vi "solar_misc CPU Usage.vi"(8 "error in (no error)":errorcluster, 9 "Close Refnums? (F)":bool) -> (0 "error out":errorcluster, 2 "Processor CPU Usage (%)":dbl[](array[numeric]), 3 "Total CPU Usage (%)":dbl)   [LabVIEW 2018]
doc: "This returns the CPU utilization in percent for each processor using the .NET System.Diagnostics.PerformanceCounter API."
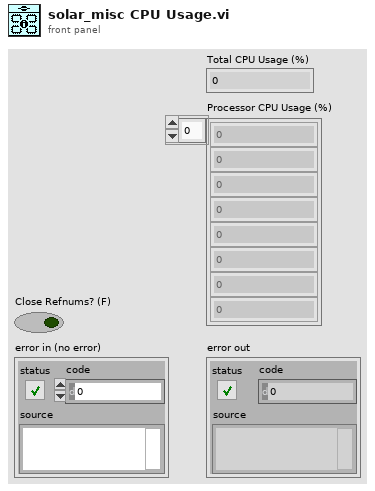
[diagram p1: front panel]
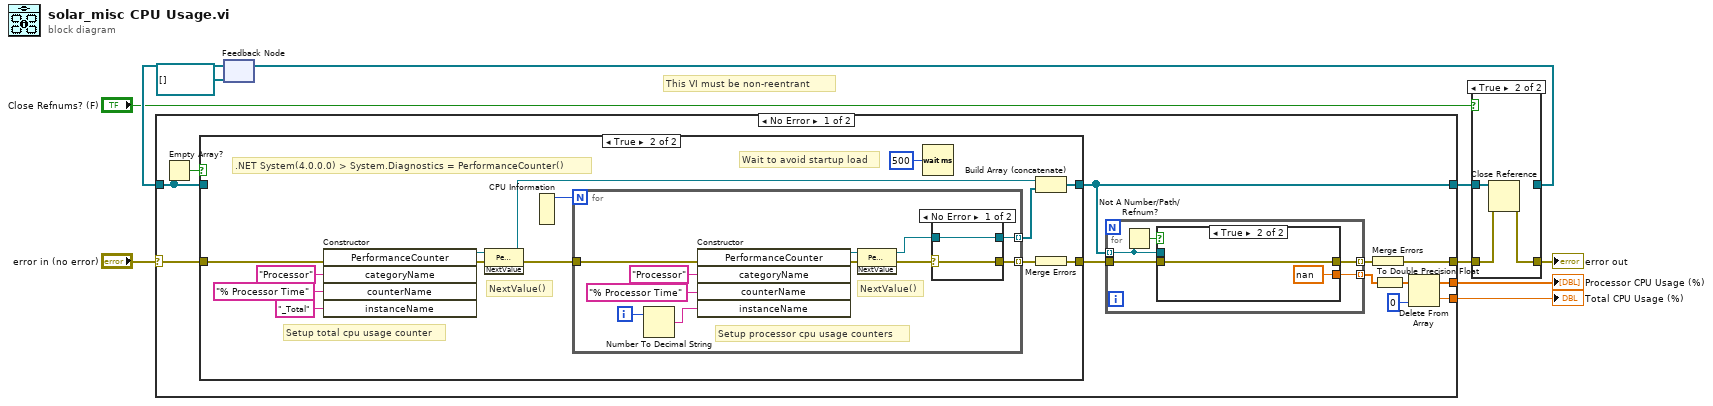
[diagram p0: block diagram]
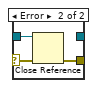
[diagram p4: hidden frame]
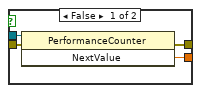
[diagram p5: hidden frame]
diagram:
  # "This VI must be non-reentrant"
  n1 = feedback #1(refnum<k24>[] []) -> (w10:refnum<k24>[])
  n2 = case shown="No Error" "error in (no error)" {
    selector: "error in (no error)" -> [w22 w67]
    tunnel: [w18 w66] -> w3
    tunnel: w10 -> [w21 w66]
    tunnel: [w16 w67] -> w5
    tunnel: [w13 _] -> w7
    tunnel: [w12 _] -> w6
    frame No Error {
      n3 = Empty Array?(array=w21) -> (empty?=w20:bool)
      n4 = case shown="True" w20 {
        tunnel: [w24 w33] -> w18
        tunnel: w21 -> [w24 _]
        tunnel: w22 -> [w23 w31]
        tunnel: [w23 w30] -> w19
        frame False {
        }
        frame True {
          # "Wait to avoid startup load"
          # "Setup total cpu usage counter"
          # "NextValue()"
          # ".NET System(4.0.0.0) > System.Diagnostics = PerformanceCounter()"
          n5 = constructor class="PerformanceCounter"(error in=w31, "categoryName"="Processor", "counterName"="% Processor Time", "instanceName"="_Total") -> (reference out=w28:refnum<k24>, error out=w29:errorcluster)  [unwired: 2 in, 4 out]
          n6 = invoke class="PerformanceCounter" method="NextValue"(reference=w28, error in=w29) -> (reference out=w26:refnum<k24>, error out=w27:errorcluster)  [unwired: 1 in, 1 out]
          n7 = CPU Information() -> (4:w38:i32)  [unwired: 3 out]
          n8 = for {
            N: w38 -> [_]
            tunnel: [w40] -> w37 mode=indexing
            tunnel: [w39] -> w32 mode=indexing
            tunnel: w27 -> [w43]
            i -> [w45]
            # "Setup processor cpu usage counters"
            # "NextValue()"
            n9 = Number To Decimal String(number=w45) -> (decimal integer string=w44:string)  [unwired: 1 in]
            n10 = constructor class="PerformanceCounter"(error in=w43, "categoryName"="Processor", "counterName"="% Processor Time", "instanceName"=w44) -> (reference out=w48:refnum<k24>, error out=w49:errorcluster)  [unwired: 2 in, 4 out]
            n11 = invoke class="PerformanceCounter" method="NextValue"(reference=w48, error in=w49) -> (reference out=w42:refnum<k24>, error out=w41:errorcluster)  [unwired: 1 in, 1 out]
            n12 = case shown="No Error" w41 {
              selector: w41 -> [w51 w53]
              tunnel: w42 -> [w50 w54]
              tunnel: [w51 w52] -> w40
              tunnel: [w50 _] -> w39
              frame No Error {
              }
              frame Error {
                n13 = Close Reference(reference=w54, error in (no error)=w53) -> (error out=w52:errorcluster)
              }
            }
          }
          n14 = Wait (ms)(milliseconds to wait=u32 500) -> ()  [unwired: 1 out]
          n15 = Build Array (concatenate)(w26, w32) -> (w33:refnum<k24>[])
          n16 = Merge Errors(w37) -> (w30:errorcluster)
        }
      }
      n17 = for {
        tunnel: w18 -> [w56] mode=indexing
        tunnel: w19 -> [w59]
        tunnel: [w58] -> w15 mode=indexing
        tunnel: [w57] -> w17 mode=indexing
        n18 = Not A Number/Path/Refnum?(number/path/refnum=w56) -> (NaN/Path/Refnum?=w55:bool)
        n19 = case shown="True" w55 {
          tunnel: w56 -> [w63 _]
          tunnel: w59 -> [w62 w65]
          tunnel: [w61 sgl nan ("NextValue")] -> w58
          tunnel: [w60 w65] -> w57
          frame False {
            n20 = invoke class="PerformanceCounter" method="NextValue"(reference=w63, error in=w62) -> (error out=w60:errorcluster, "NextValue"=w61:sgl)  [unwired: 1 in, 1 out]
          }
          frame True {
          }
        }
      }
      n21 = Merge Errors(w17) -> (w16:errorcluster)
      n22 = To Double Precision Float(number=w15) -> (double precision float=w11:dbl[])
      n23 = Delete From Array(array=w11, index=0) -> (deleted portion=w13:dbl, array with subset deleted=w12:dbl[])  [unwired: 1 in]
    }
    frame Error {
    }
  }
  "Total CPU Usage (%)" <- w7
  "Processor CPU Usage (%)" <- w6
  n24 = case shown="True" "Close Refnums? (F)" {
    tunnel: w3 -> [w69 w72]
    tunnel: [w69 _] -> w2
    tunnel: [w68 w70] -> w4
    tunnel: w5 -> [w68 w71]
    frame False {
    }
    frame True {
      n25 = Close Reference(reference=w72, error in (no error)=w71) -> (error out=w70:errorcluster)
    }
  }
  "error out" <- w4
  n26 = feedback-in #1(w2) -> ()
